vi "Prepare Testing Data.vi"() -> (2 "Attr Data":refnum<class "Tree Data.lvclass">[](array[class]), 3 "Attr Names":string[](array[string]))   [LabVIEW 2017, in "Tree API.lvlib" / "Tree.lvclass"]
uses:
  Tree.lvclass
  Tree Data/Tree Data.lvclass
  API/From Variant.vi
  Data Types/2D Flt/From 2D Float Tree Data.vi
  Data Types/2D Flt/2D Flt.lvclass
  Data Types/2D Int/From 2D Int Tree Data.vi
  Data Types/2D Int/2D Int.lvclass
  Data Types/Int Array/From 1D Int Tree Data.vi
  Data Types/Int Array/1D Int.lvclass
  Data Types/Flt Array/From 1D Float Tree Data.vi
  Data Types/Flt Array/1D Flt.lvclass
  Data Types/Int/From Integer Tree Data.vi
  Data Types/Int/Int.lvclass
  Data Types/Float/From Float Tree Data.vi
  Data Types/Float/Flt.lvclass
  Data Types/Bool Array/From 1D Bool Tree Data.vi
  Data Types/Bool Array/1D Bool.lvclass
  Data Types/2D Bool/From 2D Bool Tree Data.vi
  Data Types/2D Bool/2D Bool.lvclass
  Data Types/Bool/From Bool Tree Data.vi
  Data Types/Bool/Bool.lvclass
  API/To Variant.vi
  Data Types/2D Flt/To 2D Float Tree Data.vi
  Data Types/Flt Array/To 1D Float Tree Data.vi
  Data Types/Float/To Float Tree Data.vi
  Data Types/2D Bool/To 2D Bool Tree Data.vi
  Data Types/Bool Array/To 1D Bool Tree Data.vi
  Data Types/Bool/To Bool Tree Data.vi
  Data Types/2D Int/To 2D Int Tree Data.vi
  Data Types/Int Array/To 1D Int Tree Data.vi
  Data Types/Int/To Integer Tree Data.vi
  Data Types/Path/To Path Tree Data.vi
  Data Types/Path/Path.lvclass
  Data Types/Path Array/To 1D Path Tree Data.vi
  Data Types/Path Array/1D Path.lvclass
  Data Types/Path/From Path Tree Data.vi
  Data Types/Path Array/From 1D Path Tree Data.vi
  Data Types/2D Path/From 2D Path Tree Data.vi
  Data Types/2D Path/2D Path.lvclass
  Data Types/2D Path/To 2D Path Tree Data.vi
  Data Types/String/To String Tree Data.vi
  Data Types/String/String.lvclass
  Data Types/String Array/To 1D String Tree Data.vi
  Data Types/String Array/1D String.lvclass
  Data Types/2D String/To 2D String Tree Data.vi
  Data Types/2D String/2D String.lvclass
  Data Types/String/From String Tree Data.vi
  Data Types/String Array/From 1D String Tree Data.vi
  Data Types/2D String/From 2D String Tree Data.vi
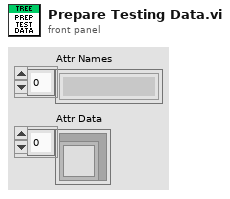
[diagram p1: front panel]
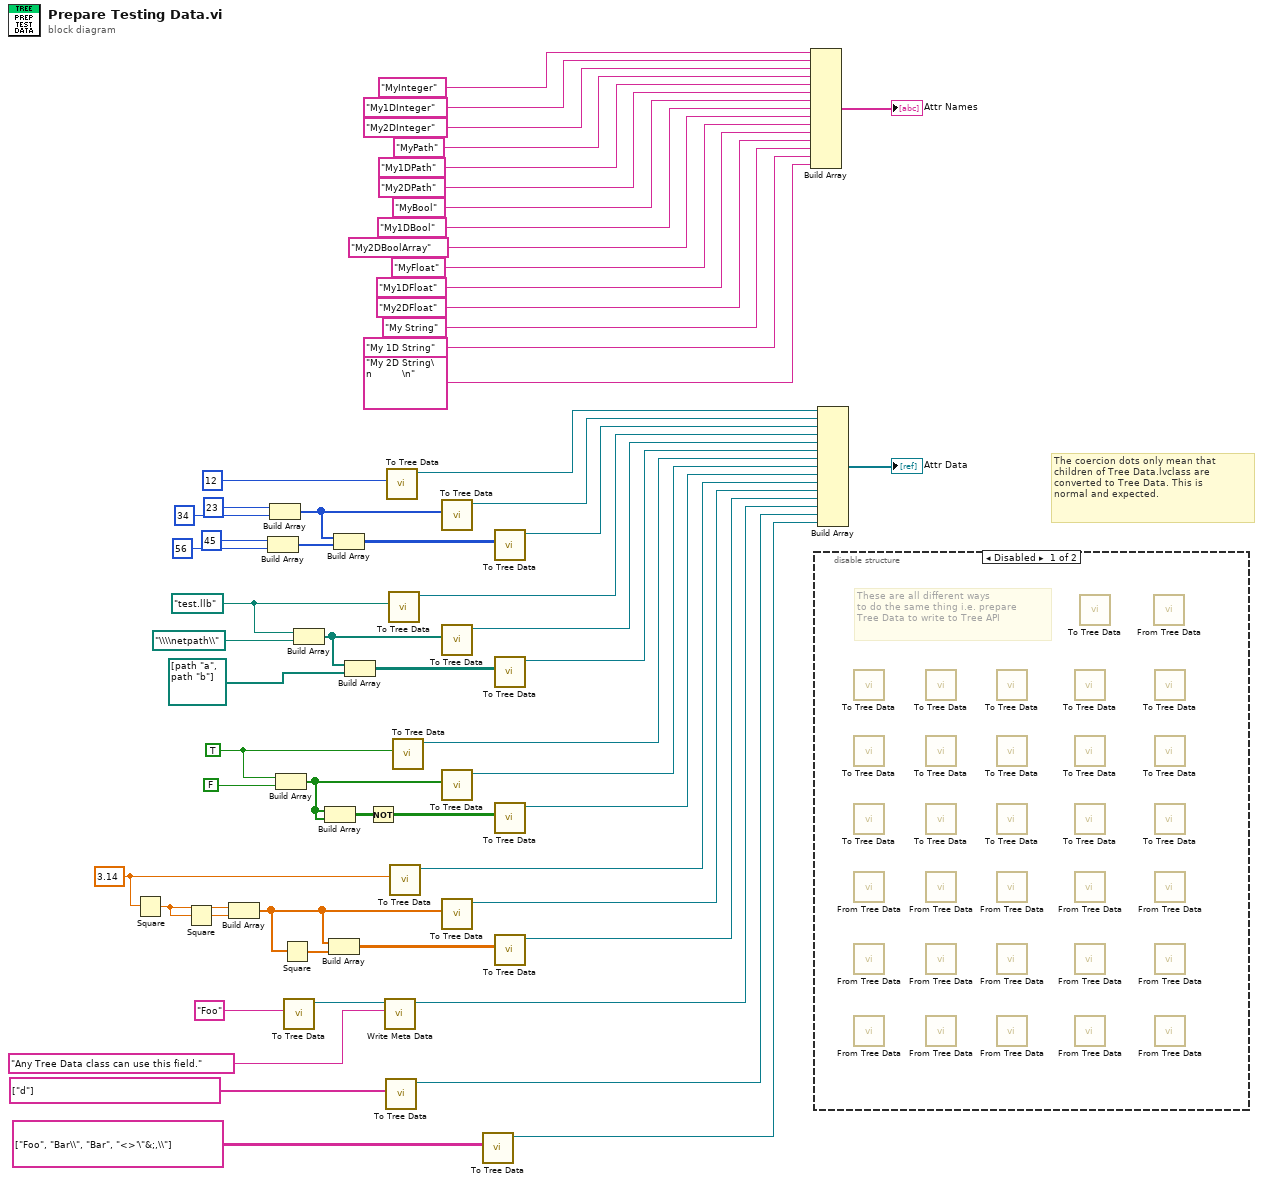
[diagram p0: block diagram]
diagram:
  w34 = 3.14 ("Float")
  w28 = TRUE ("Boolean")
  w21 = path "test.llb" ("Path")
  # "The coercion dots only mean that \nchildren of Tree Data.lvclass are\nconverted to Tree Data. This is \nnormal and expected."
  n1 = Square(x=w34) -> (x^2=w37:dbl)
  n2 = Square(x=w37) -> (x^2=w38:dbl)
  n3 = Build Array(w37, w38) -> (w32:dbl[])
  n4 = Build Array(u64 45 ("Integer"), u64 56 ("Integer")) -> (w39:u64[])
  n5 = Build Array(u64 23 ("Integer"), u64 34 ("Integer")) -> (w19:u64[])
  n6 = Build Array(w28, FALSE ("element")) -> (w25:bool[])
  n7 = Square(x=w32) -> (x^2=w36:dbl[])
  n8 = call-poly "To Tree Data.vi"("Variant"="Foo" ("String")) -> ("Tree Data Out"=w12:refnum<class "Tree Data.lvclass">)  [unwired: 9 in, 1 out]
  n9 = Build Array(w21, path "\\\\netpath\\" ("Path")) -> (w10:path[])
  n10 = Build Array(w25, w25) -> (w23:bool[][])
  n11 = Build Array(w32, w36) -> (w31:dbl[][])
  n12 = Build Array(w19, w39) -> (w17:u64[][])
  n13 = Build Array(w10, path[] [path "a", path "b"] ("element")) -> (w9:path[][])
  n14 = Not(x=w23) -> (.not. x?=w22:bool[][])
  n15 = call "Write Meta Data.vi"("Meta Data"="Any Tree Data class can use this field.", "Tree Data In"=w12) -> ("Tree Data Out"=w11:refnum<class "Tree Data.lvclass">)  [unwired: 9 in]
  n16 = call-poly "To Tree Data.vi"("Variant"=string[] ["d"] ("String Array")) -> ("Tree Data Out"=w45:refnum<class "Tree Data.lvclass">)  [unwired: 9 in, 1 out]
  n17 = call-poly "To Tree Data.vi"("Variant"=u64 12 ("Integer")) -> ("Tree Data Out"=w44:refnum<class "Tree Data.lvclass">)  [unwired: 9 in, 1 out]
  n18 = call-poly "To Tree Data.vi"("Variant"=w21) -> ("Tree Data Out"=w20:refnum<class "Tree Data.lvclass">)  [unwired: 9 in, 1 out]
  n19 = call-poly "To Tree Data.vi"("Variant"=w34) -> ("Tree Data Out"=w33:refnum<class "Tree Data.lvclass">)  [unwired: 9 in, 1 out]
  n20 = call-poly "To Tree Data.vi"("Variant"=w28) -> ("Tree Data Out"=w27:refnum<class "Tree Data.lvclass">)  [unwired: 9 in, 1 out]
  n21 = call-poly "To Tree Data.vi"("Variant"=w19) -> ("Tree Data Out"=w18:refnum<class "Tree Data.lvclass">)  [unwired: 9 in, 1 out]
  n22 = call-poly "To Tree Data.vi"("Variant"=w10) -> ("Tree Data Out"=w8:refnum<class "Tree Data.lvclass">)  [unwired: 9 in, 1 out]
  n23 = call-poly "To Tree Data.vi"("Variant"=w25) -> ("Tree Data Out"=w26:refnum<class "Tree Data.lvclass">)  [unwired: 9 in, 1 out]
  n24 = call-poly "To Tree Data.vi"("Variant"=w32) -> ("Tree Data Out"=w29:refnum<class "Tree Data.lvclass">)  [unwired: 9 in, 1 out]
  n25 = call-poly "To Tree Data.vi"("Variant"=string[][] [["Foo", "Bar\\"], ["Bar", "<>'\"&;,\\"]] ("String Array")) -> ("Tree Data Out"=w1:refnum<class "Tree Data.lvclass">)  [unwired: 9 in, 1 out]
  n26 = call-poly "To Tree Data.vi"("Variant"=w17) -> ("Tree Data Out"=w16:refnum<class "Tree Data.lvclass">)  [unwired: 9 in, 1 out]
  n27 = call-poly "To Tree Data.vi"("Variant"=w9) -> ("Tree Data Out"=w7:refnum<class "Tree Data.lvclass">)  [unwired: 9 in, 1 out]
  n28 = call-poly "To Tree Data.vi"("Variant"=w22) -> ("Tree Data Out"=w24:refnum<class "Tree Data.lvclass">)  [unwired: 9 in, 1 out]
  n29 = call-poly "To Tree Data.vi"("Variant"=w31) -> ("Tree Data Out"=w30:refnum<class "Tree Data.lvclass">)  [unwired: 9 in, 1 out]
  n30 = Build Array("MyInteger" ("Name"), "My1DInteger" ("Name"), "My2DInteger" ("Name"), "MyPath" ("Name"), "My1DPath" ("Name"), "My2DPath" ("Name"), "MyBool" ("Name"), "My1DBool" ("Name"), "My2DBoolArray" ("Name"), "MyFloat" ("Name"), "My1DFloat" ("Name"), "My2DFloat" ("Name"), "My String" ("Name"), "My 1D String" ("Name"), "My 2D String\n          \n" ("Name")) -> (→"Attr Names":string[])
  n31 = disable-structure shown="Disabled" {
    frame Disabled {
      # "These are all different ways\nto do the same thing i.e. prepare\nTree Data to write to Tree API"
      n32 = call-poly "To Tree Data.vi"() -> ()  [unwired: 11 in, 1 out]
      n33 = call-poly "To Tree Data.vi"() -> ()  [unwired: 11 in, 1 out]
      n34 = call-poly "To Tree Data.vi"() -> ()  [unwired: 11 in, 1 out]
      n35 = call-poly "From Tree Data.vi"() -> ()  [unwired: 11 in, 1 out]
      n36 = call-poly "From Tree Data.vi"() -> ()  [unwired: 11 in, 1 out]
      n37 = call-poly "From Tree Data.vi"() -> ()  [unwired: 11 in, 1 out]
      n38 = call-poly "To Tree Data.vi"() -> ()  [unwired: 11 in, 1 out]
      n39 = call-poly "To Tree Data.vi"() -> ()  [unwired: 11 in, 1 out]
      n40 = call-poly "To Tree Data.vi"() -> ()  [unwired: 11 in, 1 out]
      n41 = call-poly "From Tree Data.vi"() -> ()  [unwired: 11 in, 1 out]
      n42 = call-poly "From Tree Data.vi"() -> ()  [unwired: 11 in, 1 out]
      n43 = call-poly "From Tree Data.vi"() -> ()  [unwired: 11 in, 1 out]
      n44 = call-poly "To Tree Data.vi"() -> ()  [unwired: 11 in, 1 out]
      n45 = call-poly "To Tree Data.vi"() -> ()  [unwired: 11 in, 1 out]
      n46 = call-poly "To Tree Data.vi"() -> ()  [unwired: 11 in, 1 out]
      n47 = call-poly "From Tree Data.vi"() -> ()  [unwired: 11 in, 1 out]
      n48 = call-poly "From Tree Data.vi"() -> ()  [unwired: 11 in, 1 out]
      n49 = call-poly "From Tree Data.vi"() -> ()  [unwired: 11 in, 1 out]
      n50 = call-poly "To Tree Data.vi"() -> ()  [unwired: 11 in, 1 out]
      n51 = call-poly "To Tree Data.vi"() -> ()  [unwired: 11 in, 1 out]
      n52 = call-poly "To Tree Data.vi"() -> ()  [unwired: 11 in, 1 out]
      n53 = call-poly "From Tree Data.vi"() -> ()  [unwired: 11 in, 1 out]
      n54 = call-poly "From Tree Data.vi"() -> ()  [unwired: 11 in, 1 out]
      n55 = call-poly "From Tree Data.vi"() -> ()  [unwired: 11 in, 1 out]
      n56 = call-poly "To Tree Data.vi"() -> ()  [unwired: 10 in, 2 out]
      n57 = call-poly "From Tree Data.vi"() -> ()  [unwired: 10 in, 2 out]
      n58 = call-poly "To Tree Data.vi"() -> ()  [unwired: 11 in, 1 out]
      n59 = call-poly "To Tree Data.vi"() -> ()  [unwired: 11 in, 1 out]
      n60 = call-poly "To Tree Data.vi"() -> ()  [unwired: 11 in, 1 out]
      n61 = call-poly "From Tree Data.vi"() -> ()  [unwired: 11 in, 1 out]
      n62 = call-poly "From Tree Data.vi"() -> ()  [unwired: 11 in, 1 out]
      n63 = call-poly "From Tree Data.vi"() -> ()  [unwired: 11 in, 1 out]
    }
    frame Enabled {
    }
  }
  n64 = Build Array(w44, w18, w16, w20, w8, w7, w27, w26, w24, w33, w29, w30, w11, w45, w1) -> (→"Attr Data":refnum<class "Tree Data.lvclass">[])
